vi "OAT Extract Slow Roll Vectors (Single Channel).vi"(5 "reset? (True)":bool=TRUE, 6 "max order (auto)":i32, 7 "orders (1.0)":dbl[](array[numeric])=[1.0] format="%.2f", 8 "error in (no error)":errorcluster, 9 "pulse/revolution (1)":i32=1, 10 "speed profile":T1 {"speed [RPM]" format="%.2f"; "time [s]" format="%.2f"}, 11 "scaled signal [EU]":waveform(dbl)={"t0"=timestamp(0 s since 1904-01-01), "dt"=0.0, "Y"=[]}) -> (0 "error out":errorcluster, 3 "slow roll vectors":cdb[](array[numeric]) format="%.2f")   [LabVIEW 2017]
doc: "Extract the vectors of the specified orders from the slow roll vibration signals. The vectors are used for proximity probe signals to perform run out compensation."
uses:
  <vilib>/addons/Sound and Vibration/Order Analysis/Tach Process/SubVIs/speed profile.ctl
  <vilib>/Analysis/baseanly.llb/Mean (DBL).vi
  <vilib>/addons/Sound and Vibration/Order Analysis/Resample Order Tracking/OAT Order Magnitude and Phase (Even Angle Signal, 1 Channel).vi
  <vilib>/addons/Sound and Vibration/Order Analysis/Resample Order Tracking/OAT Convert to Even Angle Signal (1 Channel).vi
  <vilib>/Analysis/NI_AALPro.lvlib
  <vilib>/addons/Sound and Vibration/Order Analysis/Resample Order Tracking/SoundVib_OrderTracking.lvlib
  <vilib>/Analysis/NI_AALBase.lvlib
  <vilib>/addons/Sound and Vibration/Order Analysis/Tach Process/SoundVib_TachProcess.lvlib
panel:
  in  "bandwidth [order]":dbl format="%.2f"
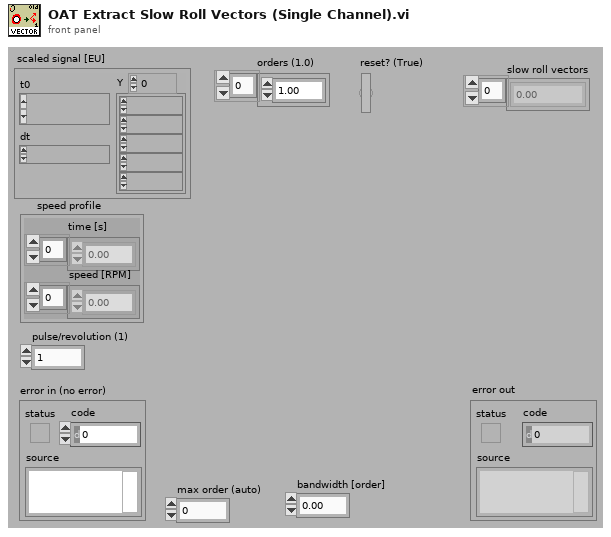
[diagram p1: front panel]
types:
  T1 = typedef "SoundVib_TachProcess.lvlib/speed profile.ctl" = cluster{"time [s]":dbl[], "speed [RPM]":dbl[]}
  T2 = cluster{"dB on? (T)":bool, "unwrap phase? (T)":bool, "unit in degree? (T)":bool}
  T3 = typedef "svc_Resampled Channel Info.ctl" = cluster{"channel name":string, "description":string, " channel info":T4}
  T4 = typedef "svc_Channel Info.ctl" = cluster{"sensor sensitivity":dbl, "engineering units":T5, "dB reference":dbl, "custom label":string, "weighting filter":T6, "pregain":dbl}
  T5 = typedef "svc_Engineering Units Text Ring.ctl" = u16
  T6 = typedef "svc_Weighting Filter Text Ring.ctl" = u16
  T7 = typedef "OAT Position Info.ctl" = cluster{"positions [s]":dbl[], "samples/rev":dbl}
  T8 = cluster{"time/rev/rpm":dbl[], "magnitude":dbl[]}[]
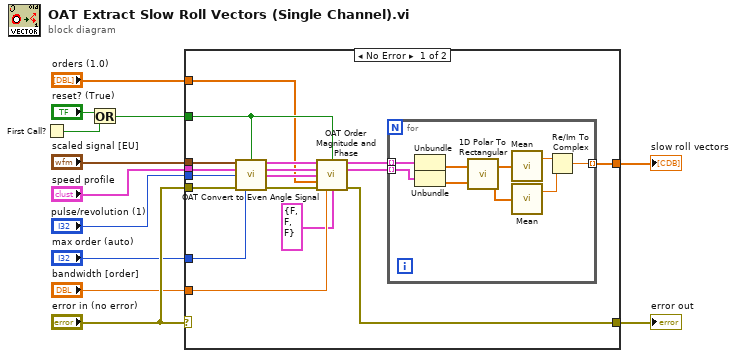
[diagram p0: block diagram]
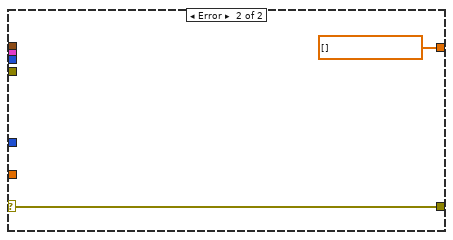
[diagram p2: hidden frame]
diagram:
  n1 = First Call?() -> (First Call?: T/F=w5:bool)
  n2 = Or(x="reset? (True)", y=w5) -> (x .or. y?=w4:bool)
  n3 = case shown="No Error" "error in (no error)" {
    selector: "error in (no error)" -> [_ w39]
    tunnel: "scaled signal [EU]" -> [w29 _]
    tunnel: "speed profile" -> [w28 _]
    tunnel: "pulse/revolution (1)" -> [w27 _]
    tunnel: "error in (no error)" -> [w26 _]
    tunnel: [w19 cdb[] []] -> w8
    tunnel: [w18 w39] -> w7
    tunnel: w4 -> [w16 _]
    tunnel: "max order (auto)" -> [w17 _]
    tunnel: "orders (1.0)" -> [w15 _]
    tunnel: "bandwidth [order]" -> [w14 _]
    frame No Error {
      n4 = call-poly <vilib>:"OAT Convert to Even Angle Signal.vi"("scaled signal [EU]"=w29, "reset? (F)"=w16, "speed profile"=w28, "pulse/revolution (1)"=w27, "error in (no error)"=w26, "max order (auto)"=w17) -> ("even-angle signal"=w25:cluster{"r0":dbl, "dr":dbl, "Y":dbl[]}, "even-angle channel info"=w24:T3, "even-angle position info"=w23:T7, "error out"=w22:errorcluster)  [unwired: 5 in, 1 out]
      n5 = call-poly <vilib>:"OAT Order Magnitude and Phase.vi"("even-angle signal"=w25, "reset? (F)"=w16, "even-angle channel info"=w24, "even-angle position info"=w23, "orders to compute (1.0)"=w15, "error in (no error)"=w22, "bandwidth [order]"=w14, "view"=T2 {"dB on? (T)"=FALSE, "unwrap phase? (T)"=FALSE, "unit in degree? (T)"=FALSE}) -> ("magnitudes [RMS]"=w21:T8, "phases [phase lag]"=w20:cluster{"time/rev/rpm":dbl[], "phase":dbl[]}[], "error out"=w18:errorcluster)  [unwired: 2 in, 3 out]
      n6 = for {
        tunnel: w21 -> [w38] mode=indexing
        tunnel: w20 -> [w37] mode=indexing
        tunnel: [w31] -> w19 mode=indexing
        n7 = Unbundle(w38) -> ("magnitude"=w36:dbl[])  [unwired: 1 out]
        n8 = Unbundle(w37) -> ("phase"=w30:dbl[])  [unwired: 1 out]
        n9 = call <vilib>:"1D Polar To Rectangular.vi"("Magnitude"=w36, "Phase"=w30) -> ("X"=w35:dbl[], "Y"=w34:dbl[])  [unwired: 1 out]
        n10 = call-poly <vilib>:"Mean.vi"("X"=w35) -> ("mean"=w33:dbl)  [unwired: 1 out]
        n11 = call-poly <vilib>:"Mean.vi"("X"=w34) -> ("mean"=w32:dbl)  [unwired: 1 out]
        n12 = Re/Im To Complex(1:w32, 2:w33) -> (0:w31:cdb)
      }
    }
    frame Error {
    }
  }
  "error out" <- w7
  "slow roll vectors" <- w8
